vi "niScope Actual Num Wfms.vi"(8 "error in":errorcluster, 10 "channels":string="0", 11 "instrument handle":refnum<k15>) -> (0 "error out":errorcluster, 2 "actual num wfms":i32, 3 "instrument handle out":refnum<k15>)   [LabVIEW 2013]
doc: "Allows you to declare appropriately sized waveforms. NI-SCOPE handles the channel list parsing for you."
uses:
  niScope_32.dll
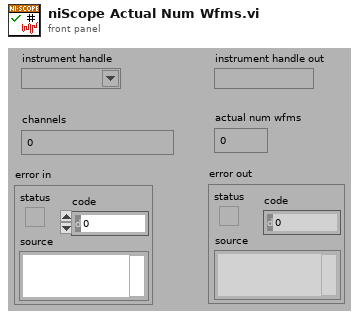
[diagram p1: front panel]
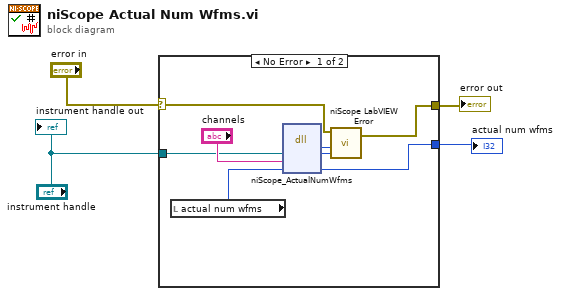
[diagram p0: block diagram]
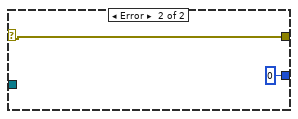
[diagram p2: hidden frame]
diagram:
  n1 = case shown="No Error" "error in" {
    selector: "error in" -> [w5 w13]
    tunnel: [w10 w13] -> w4
    tunnel: [w6 0 ("numWaveforms")] -> w3
    tunnel: "instrument handle" -> [w8 _]
    frame No Error {
      n2 = local read "actual num wfms"() -> (w7:i32)
      n3 = dll-call lib="niScope_*.*" fn="niScope_ActualNumWfms"("instrument handle"=w8, "channelList"="channels", "numWfms"=w7) -> ("status"=w12:i32, "instrument handle"=w11:u32, "numWfms"=w6:i32)  [unwired: 4 in, 2 out]
      n4 = call <instrlib>:"niScope LabVIEW Error.vi"("instrument handle"=w11, "niScope error code (0)"=w12, "error in (no error)"=w5) -> ("error out"=w10:errorcluster)  [unwired: 2 in]
    }
    frame Error {
    }
  }
  "actual num wfms" <- w3
  "error out" <- w4
  "instrument handle out" <- "instrument handle"
